vi "Set Acquisition Registers.vi"(0 "acq in":refnum<class "niUSRP Rx DSP v2 FPGA.lvclass">, 5 "acq registers":refnum<class "Address Space Collection.lvclass">) -> (4 "acq out":refnum<class "niUSRP Rx DSP v2 FPGA.lvclass">)   [LabVIEW 2025, in "niUSRP Rx DSP v2 FPGA.lvclass"]
doc: "this VI is an Acquisition class accessor for private data."
uses:
  niUSRP Rx DSP v2 FPGA.lvclass
  <instrlib>/_niInstr/Instruction Framework/v1/FPGA/Interfaces/Address Space Collection/Address Space Collection.lvclass
  niUSRP Rx DSP v2 FPGA.lvclass/niUSRP Rx DSP v2 FPGA.ctl
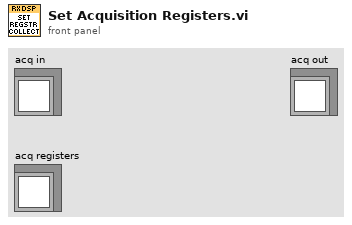
[diagram p1: front panel]
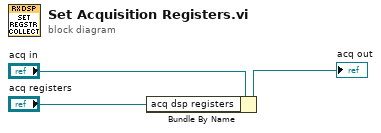
[diagram p0: block diagram]
diagram:
  n1 = Bundle By Name(cluster="acq in", "acq dsp registers"="acq registers") -> (→"acq out":refnum<class "niUSRP Rx DSP v2 FPGA.lvclass">)
